vi "Save JSON File.vi"(8 "error in (no error)":errorcluster, 10 "Data":variant, 11 "Control Experiment in":refnum<class "Control Experiment.lvclass">) -> (0 "error out":errorcluster)   [LabVIEW 2016, in "Control Experiment.lvclass"]
uses:
  Control Experiment.lvclass
  Control Experiment.lvclass/Control Experiment.ctl
  <vilib>/addons/_JKI.lib/Serialization/JSON/JKI JSON Serialization.lvlib
panel:
  out "Control Experiment out":refnum<class "Control Experiment.lvclass">
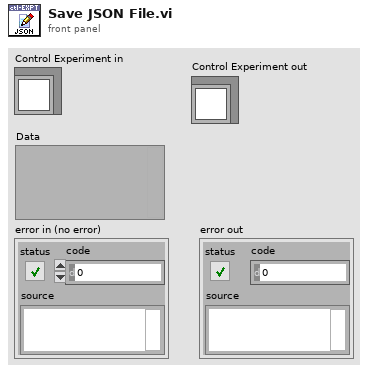
[diagram p1: front panel]
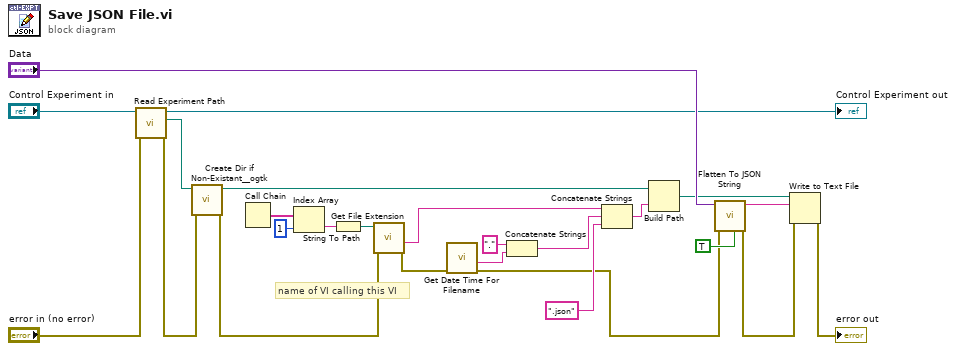
[diagram p0: block diagram]
diagram:
  # "name of VI calling this VI"
  n1 = call "Read Experiment Path.vi"("error in (no error)"="error in (no error)", "Control Experiment in"="Control Experiment in") -> ("error out"=w16:errorcluster, "Experiment Path"=w12:path, "Control Experiment out"=→"Control Experiment out":refnum<class "Control Experiment.lvclass">)  [unwired: 7 in]
  n2 = call <userlib>:"Create Dir if Non-Existant__ogtk.vi"("error in (no error)"=w16, "Directory Path"=w12) -> ("error out"=w7:errorcluster, "dup Directory Path"=w1:path)  [unwired: 7 in, 1 out]
  n3 = Call Chain() -> (call chain=w22:string[])
  n4 = Index Array(array=w22, index=1) -> (element=w23:string)
  n5 = String To Path(string=w23) -> (path=w25:path)
  n6 = call <vilib>:"Get File Extension.vi"("error in (no error)"=w7, "file"=w25) -> ("error out"=w8:errorcluster, "filename without extension"=w5:string)  [unwired: 5 in, 3 out]
  n7 = call "Get Date Time For Filename.vi"("error in (no error)"=w8) -> ("error out"=w6:errorcluster, "date-time string"=w3:string)  [unwired: 8 in, 1 out]
  n8 = Concatenate Strings("." ("string"), w3) -> (w2:string)
  n9 = Concatenate Strings(w5, w2, ".json" ("string")) -> (w20:string)
  n10 = Build Path(base path=w1, name or relative path=w20) -> (appended path=w11:path)
  n11 = call <vilib>:"Flatten To JSON String.vi"("Enums As String (F)"=TRUE, "error in (no error)"=w6, "Variant"="Data") -> ("error out"=w15:errorcluster, "JSON String"=w19:string)  [unwired: 7 in]
  n12 = Write to Text File(file (use dialog)=w11, text=w19, error in=w15) -> (error out=→"error out":errorcluster)  [unwired: 1 in, 2 out]
